vi "配置读取.vi"(8 "error in (no error)":errorcluster) -> (0 "error out":errorcluster)   [LabVIEW 2022 SP3, in "斯坦道多参数.lvlib"]
uses:
  <vilib>/Utility/config.llb/NI_LVConfig.lvlib
  <userlib>/_OpenG.lib/variantconfig/variantconfig.llb/openg_variant_configuration_file.lvlib
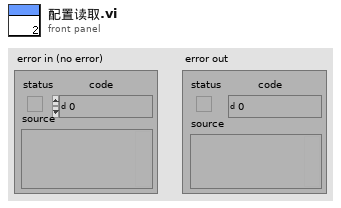
[diagram p1: front panel]
types:
  T1 = typedef "NI_LVConfig.lvlib/Config Data RefNum.ctl" = refnum<k1>
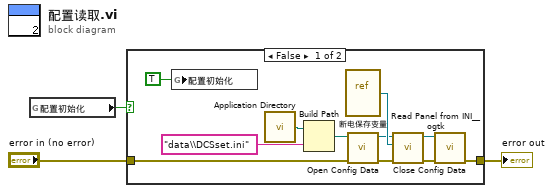
[diagram p0: block diagram]
diagram:
  n1 = global read "多参数全局变量.vi" "配置初始化"() -> (w1:bool)
  n2 = case shown="False" w1 {
    tunnel: "error in (no error)" -> [w6 w15]
    tunnel: [w5 w15] -> w2
    frame False {
      n3 = global write "多参数全局变量.vi" "配置初始化"(TRUE ("配置初始化")) -> ()
      n4 = call <vilib>:"Application Directory.vi"() -> ("Application Directory"=w13:path)
      n5 = Build Path(base path=w13, name or relative path="data\\DCSset.ini" ("名称或相对路径")) -> (appended path=w14:path)
      n6 = vi-ref "断电保存变量.vi"() -> (w11:refnum<vi>)
      n7 = call <vilib>:"Open Config Data.vi"("error in (no error)"=w6, "configuration file path"=w14) -> ("error out"=w8:errorcluster, "refnum"=w7:T1)  [unwired: 7 in, 1 out]
      n8 = call <userlib>:"Read Panel from INI__ogtk.vi"("error in (no error)"=w8, "VI ref"=w11, "refnum"=w7) -> ("error out"=w10:errorcluster, "refnum out"=w9:T1)  [unwired: 7 in]
      n9 = call <vilib>:"Close Config Data.vi"("error in (no error)"=w10, "refnum"=w9) -> ("error out"=w5:errorcluster)  [unwired: 8 in, 1 out]
    }
    frame True {
    }
  }
  "error out" <- w2
